vi "Collision Main.vi"() -> (2 "Level of Collision":dbl)   [LabVIEW 2016]
uses:
  <vilib>/Rock Robotics/Network Tables/SD Write Boolean.vi
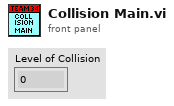
[diagram p1: front panel]
types:
  T1 = cluster{"LinearAcceleration X":dbl, "LinearAcceleration Y":dbl, "LinearAcceleration Z":dbl}
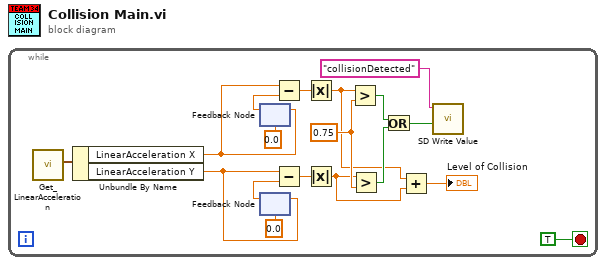
[diagram p0: block diagram]
diagram:
  n1 = while {
    stop <- TRUE stop-if-true
    w9 = 0.75
    n2 = call <vilib>:"Get_LinearAcceleration.vi"() -> ("Linear Acceleration"=w1:T1)  [unwired: 11 in]
    n3 = Unbundle By Name(w1) -> ("LinearAcceleration X"=w15:dbl, "LinearAcceleration Y"=w8:dbl)
    n4 = feedback #1(0.0) -> (w16:dbl)
    n5 = feedback-in #1(w15) -> ()
    n6 = feedback #2(0.0) -> (w14:dbl)
    n7 = feedback-in #2(w8) -> ()
    n8 = Subtract(x=w15, y=w16) -> (x-y=w17:dbl)
    n9 = Subtract(x=w8, y=w14) -> (x-y=w13:dbl)
    n10 = Absolute Value(x=w17) -> (abs(x)=w5:dbl)
    n11 = Absolute Value(x=w13) -> (abs(x)=w4:dbl)
    n12 = Greater?(x=w5, y=w9) -> (0:w11:bool)
    n13 = Greater?(x=w4, y=w9) -> (0:w10:bool)
    n14 = Or(x=w11, y=w10) -> (x .or. y?=w6:bool)
    n15 = Add(x=w5, y=w4) -> (x+y=→"Level of Collision":dbl)
    n16 = call-poly <vilib>:"SD Write Value.vi"("Boolean"=w6, "Name"="collisionDetected") -> ()  [unwired: 8 in, 2 out]
  }
